vi "DeleteQueue.vi"(0 "Program Interface in":refnum<class "Program Interface.lvclass">, 4 "Queue Index":i32, 5 "error in (no error)":errorcluster) -> (14 "Program Interface out":refnum<class "Program Interface.lvclass">, 19 "error out":errorcluster)   [LabVIEW 2019, in "Program Interface.lvclass"]
uses:
  Program Interface.lvclass
  Program Interface.lvclass/Program Interface.ctl
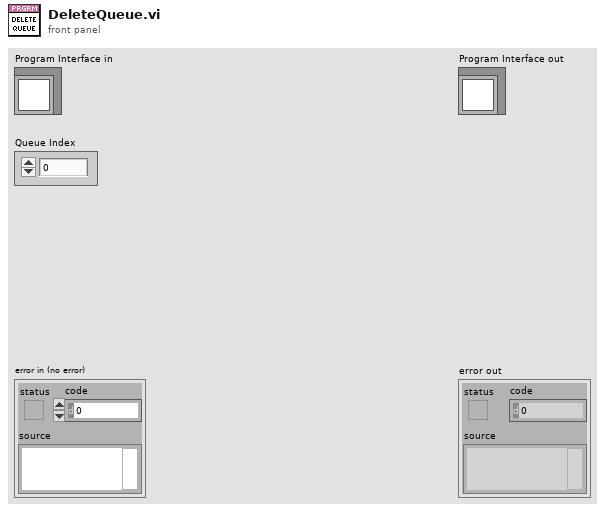
[diagram p1: front panel]
types:
  T1 = typedef "Program Interface.lvclass/SavedQueue.ctl" = cluster{"Name":string, "Programs":string[]}
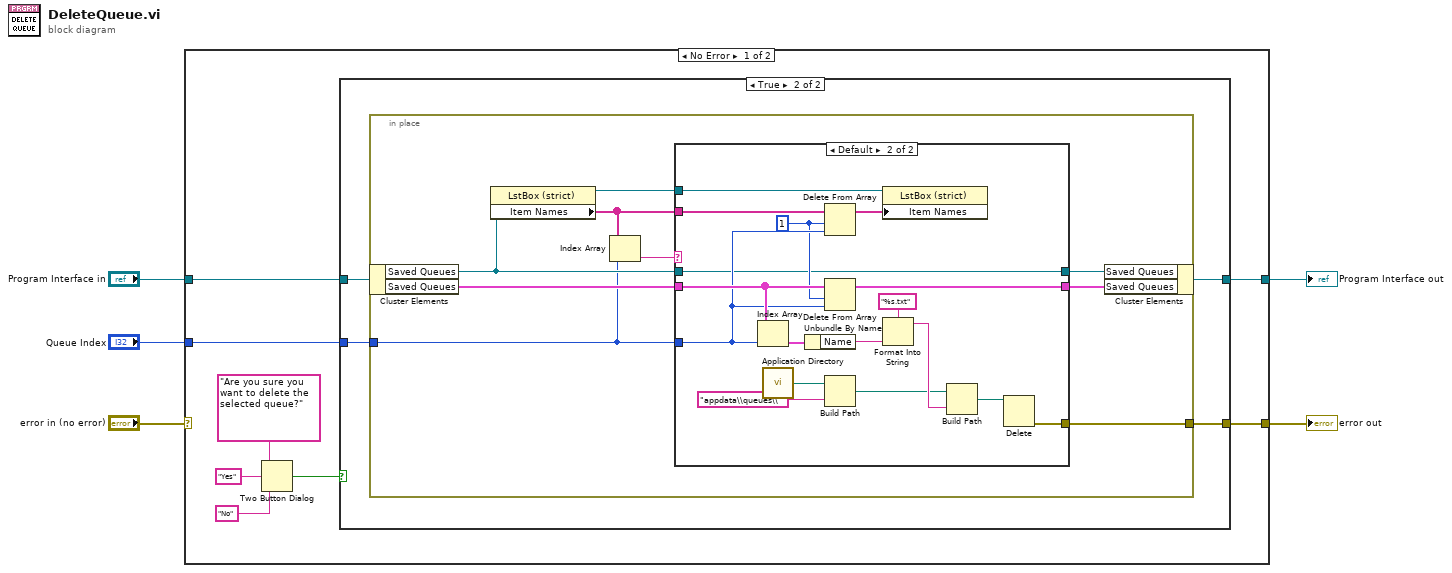
[diagram p0: block diagram]
diagram:
  n1 = case shown="No Error" "error in (no error)" {
    selector: "error in (no error)" -> [_ w48]
    tunnel: [w13 w48] -> w4
    tunnel: [w11 w47] -> w2
    tunnel: "Program Interface in" -> [w12 w47]
    tunnel: "Queue Index" -> [w10 _]
    frame No Error {
      n2 = Two Button Dialog(message="Are you sure you want to delete the selected queue?" ("T button name (\"OK\")"), 1:"No" ("F button name (\"Cancel\")"), 2:"Yes" ("T button name (\"OK\")")) -> (T button?=w9:bool)
      n3 = case shown="True" w9 {
        tunnel: [_ w18] -> w13
        tunnel: w12 -> [w14 w17]
        tunnel: [w14 w16] -> w11
        tunnel: w10 -> [_ w15]
        frame False {
        }
        frame True {
          n4 = in-place {
            in-place-border: [w25] -> w18
            in-place-border: w15 -> [w19]
            n5 = in-place-cluster #1(w17) -> ("Saved Queues"=w23:refnum<vi>, "Saved Queues"=w27:T1[])
            n6 = property class="LstBox (strict)"(reference=w23) -> (reference out=w24:refnum<vi>, "Item Names"=w21:string[])  [unwired: 1 in, 1 out]
            n7 = Index Array(array=w21, index=w19) -> (element=w20:string)
            n8 = case shown="Default" w20 {
              tunnel: w27 -> [w28 w38]
              tunnel: [w28 w35] -> w26
              tunnel: [_ w31] -> w25
              tunnel: w24 -> [_ w41]
              tunnel: w21 -> [_ w42]
              tunnel: w23 -> [w29 w34]
              tunnel: [w29 w34] -> w22
              tunnel: w19 -> [_ w37]
              frame "" {
              }
              frame Default {
                w36 = 1 ("length")
                n9 = Index Array(array=w38, index=w37) -> (element=w39:T1)
                n10 = call <vilib>:"Application Directory.vi"() -> ("Application Directory"=w46:path)
                n11 = Unbundle By Name(w39) -> ("Name"=w30:string)
                n12 = Delete From Array(array=w42, length=w36, index=w37) -> (array with subset deleted=w40:string[])  [unwired: 1 out]
                n13 = Delete From Array(array=w38, length=w36, index=w37) -> (array with subset deleted=w35:T1[])  [unwired: 1 out]
                n14 = Build Path(base path=w46, name or relative path="appdata\\queues\\") -> (appended path=w33:path)
                n15 = property class="LstBox (strict)"(reference=w41, "Item Names"=w40) -> ()  [unwired: 1 in, 2 out]
                n16 = Format Into String(format string="%s.txt", w30) -> (resulting string=w43:string)  [unwired: 2 in, 1 out]
                n17 = Build Path(base path=w33, name or relative path=w43) -> (appended path=w32:path)
                n18 = Delete(path (use dialog)=w32) -> (error out=w31:errorcluster)  [unwired: 4 in, 2 out]
              }
            }
            n19 = in-place-cluster #1("Saved Queues"=w22, "Saved Queues"=w26) -> (w16:refnum<class "Program Interface.lvclass">)
          }
        }
      }
    }
    frame Error {
    }
  }
  "error out" <- w4
  "Program Interface out" <- w2
